vi "List Entries.vi"(0 "BroadcastRegistry In":T1) -> (4 "BroadcastRegistry Out":T1, 6 "Array":string[](array[string]))   [LabVIEW 2017, in "Communicable State Machine.lvlib"]
doc: "### List Entries.vi\n\n-- <b>Controls</b> --\n- <b>BroadcastRegistry in</b>:\n\n-- <b>Indicators</b> --\n- <b>BroadcastRegistry out</b>:\n- <b>Array</b>:"
uses:
  Communicable State Machine.lvlib
  BroadcastRegistry.ctl
  BroadcastRegistry-Value.ctl
  AdvanceAPI/CSM - Broadcast Message Type.ctl
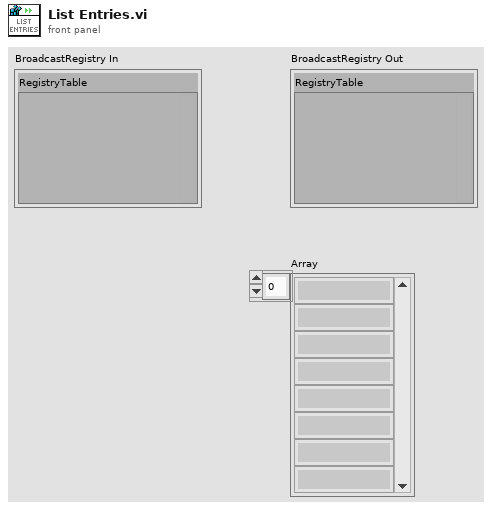
[diagram p1: front panel]
types:
  T1 = typedef "Communicable State Machine.lvlib/BroadcastRegistry.ctl" = cluster{"RegistryTable":variant}
  T2 = typedef "Communicable State Machine.lvlib/BroadcastRegistry-Value.ctl" = cluster{"Name":string, "Priority":T3}
  T3 = typedef "Communicable State Machine.lvlib/CSM - Broadcast Message Type.ctl" = enum16{"Status", "Interrupt"}
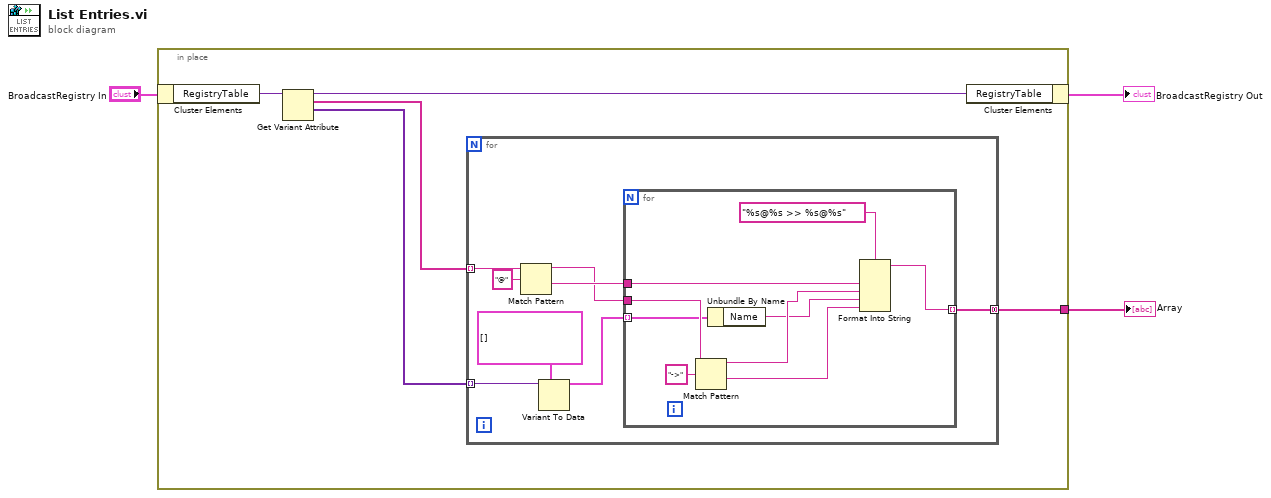
[diagram p0: block diagram]
diagram:
  n1 = in-place {
    in-place-border: [w4] -> w1
    n2 = in-place-cluster #1("BroadcastRegistry In") -> ("RegistryTable"=w8:variant)
    n3 = Get Variant Attribute(Variant=w8) -> (duplicate Variant=w7:variant, names=w5:string[], values=w6:variant[])  [unwired: 3 in, 1 out]
    n4 = for {
      tunnel: w6 -> [w16] mode=indexing
      tunnel: w5 -> [w14] mode=indexing
      tunnel: [w9] -> w4 mode=concatenating
      n5 = Match Pattern(string=w14, regular expression="@") -> (before substring=w11:string, after substring=w12:string)  [unwired: 1 in, 2 out]
      n6 = Variant To Data(type=T2[] [], Variant=w16) -> (data=w10:T2[])  [unwired: 1 in, 1 out]
      n7 = for {
        tunnel: w12 -> [w22]
        tunnel: w11 -> [w25]
        tunnel: w10 -> [w20] mode=indexing
        tunnel: [w18] -> w9 mode=indexing
        n8 = Match Pattern(string=w25, regular expression="->") -> (before substring=w21:string, after substring=w19:string)  [unwired: 1 in, 2 out]
        n9 = Unbundle By Name(w20) -> ("Name"=w17:string)
        n10 = Format Into String(format string="%s@%s >> %s@%s", w22, w21, w17, w19) -> (resulting string=w18:string)  [unwired: 2 in, 1 out]
      }
    }
    n11 = in-place-cluster #1("RegistryTable"=w7) -> (→"BroadcastRegistry Out":T1)
  }
  "Array" <- w1
